vi "Array understanding.vi"() -> ()   [LabVIEW 2019]
panel:
  out "element":dbl
  in  "Array":dbl[](array[numeric])
  out "size(s)":i32
  # "Array Uses and Indexing"
  # "2"
  # "1"
  # "3"
  # "4"
  # "0"
  # "5"
  # "6"
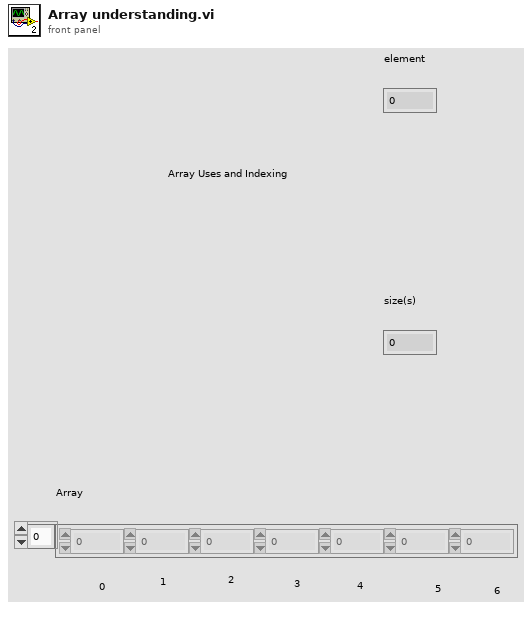
[diagram p1: front panel]
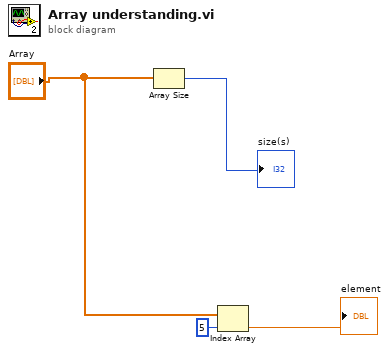
[diagram p0: block diagram]
diagram:
  n1 = Array Size(array="Array") -> (size(s)=→"size(s)":i32)
  n2 = Index Array(array="Array", index=5) -> (element=→"element":dbl)
